vi "Host 9159 cRIO Interface.vi"(10 "Number of Elements":u32=64) -> (2 "AI Data":i32[](array[numeric]))   [LabVIEW 2017]
uses:
  <vilib>/FPGAPlugInAG/NI 9159/niLvFpga_Open_NI 9159.vi
  <vilib>/rvi/interface/common/dynamic/niFpgaDynamicAddResources.vi
  <vilib>/FPGAPlugInAG/Dynamic/niLvFpga_Run_Dynamic.vi
  <vilib>/rvi/interface/common/niFpgaWaitOnOcc.vi
  <vilib>/Utility/error.llb/Error Cluster From Error Code.vi
  <vilib>/rvi/errors/niLvFpgaAdjustHostInterfaceError.vi
  <vilib>/FPGAPlugInAG/Dynamic/niLvFpga_Close_Dynamic.vi
  <vilib>/rvi/interface/nirviOpenFPGA/nirviOpenFPGA.xnode
  FPGA Bitfiles/RIOExpansionLate_FPGATarget2_9159FPGADMATop_ueHRLpdidM4.lvbitx
  FPGA/MXIe 9159 FPGA VI.vi
  <vilib>/rvi/interface/nirviMethod/nirviMethod.xnode
  <vilib>/rvi/interface/nirviReadWriteControl/nirviReadWriteControl.xnode
  <vilib>/rvi/interface/nirviCloseFPGA/nirviCloseFPGA.xnode
  <vilib>/FPGAPlugInAG/Dynamic/niLvFpga_ReadFifo_Dynamic.vi
  <vilib>/rvi/errors/niLvFpgaMergeErrorWithErrorCode.vi
  NiFpgaLv.dll
  <vilib>/rvi/interface/Simulation/niFpgaSimulationCallBeginRW.vi
  <vilib>/FPGAPlugInAG/Dynamic/niLvFpga_ConfigureFifo_Dynamic.vi
panel:
  out "Host Loop Duration (ms)":u32
  out "TargetToHostLoopIterCount":i32
  out "TargetToHostLoopTimedOut":bool
  out "SlowDOLoop_Duration_ticks":u32
  out "FastAILoop_Duration_ticks":u32
  out "Mod3_AI3_I32":i32
  out "Mod3_AI2_I32":i32
  out "Mod3_AI1_I32":i32
  out "Mod3_AI0_I32":i32
  out "SlowScanLoopTimedOut":bool
  out "SlowScanLoop_Duration_ticks":u32
  out "FastDI_U8":u8
  in  "Mod11_U32":u32
  in  "Mod10_U32":u32
  in  "Mod9_U32":u32
  in  "Mod7_U32":u32
  in  "SlowDOLoop_Rate_us":u32=10000
  in  "FastAILoop_Rate_us":u32=1000
  in  "SlowScanLoop_Rate_us":u32=10000
  in  "FastDO_U8":u8
  out "error out":errorcluster={"status"=TRUE, "code"=-50400, "source"="Invoke Method: FIFO.Read in Host 9159 cRIO Interface.vi"}
  in  "stop":bool
  out "Elements Remaining":u32=63
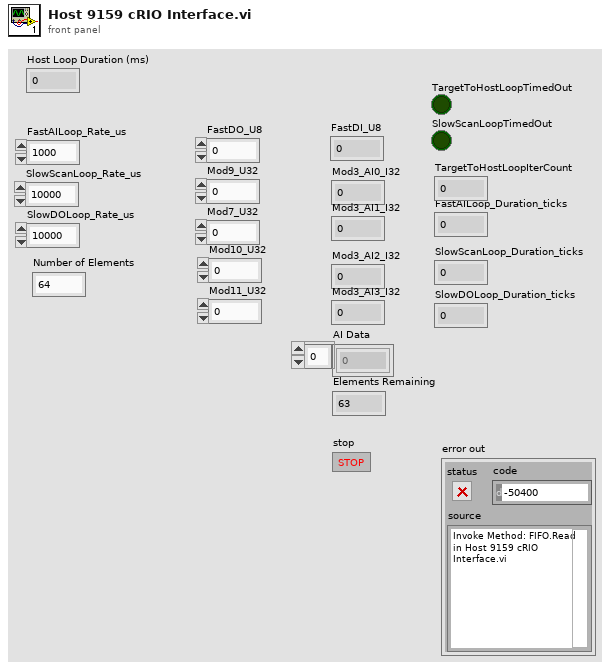
[diagram p1: front panel]
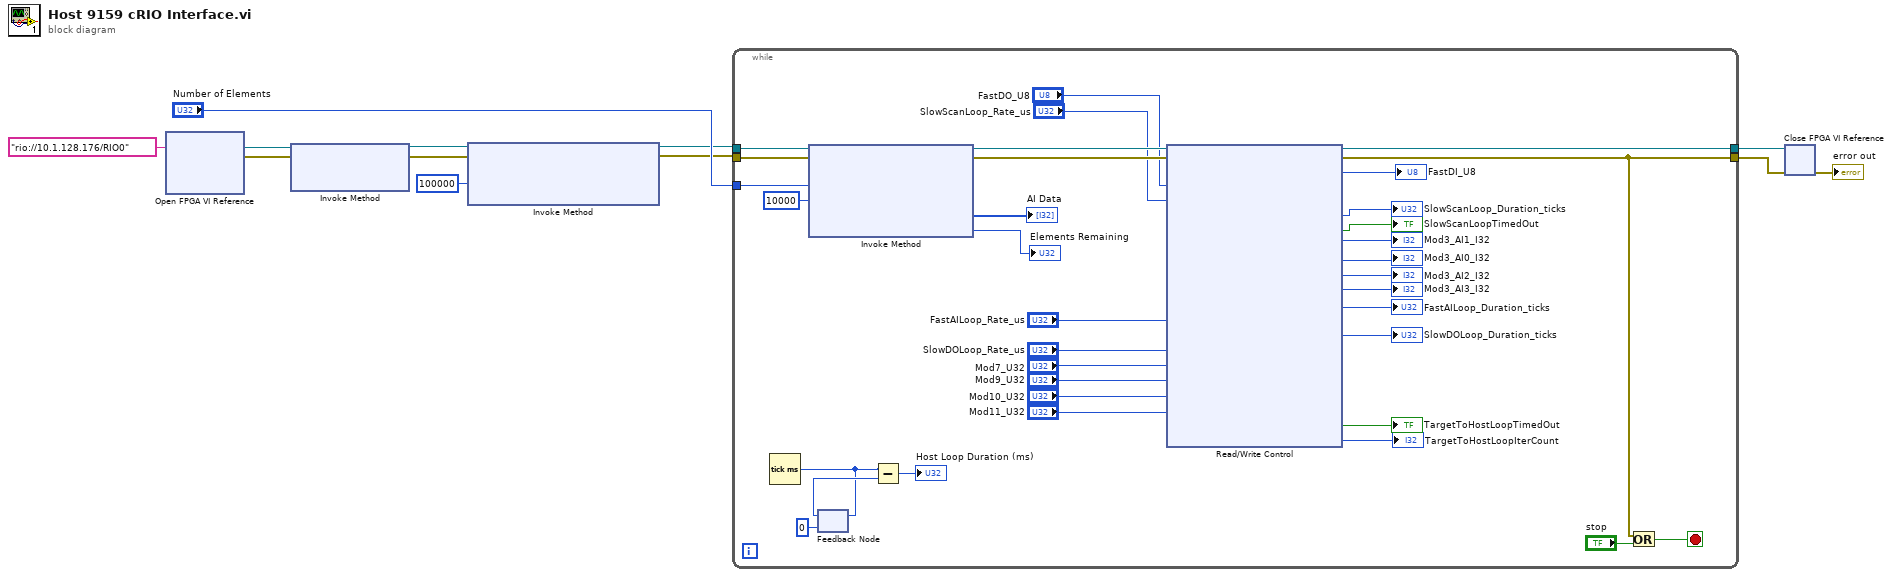
[diagram p0: block diagram]
diagram:
  n1 = xnode "Open FPGA VI Reference"("resource name"=tag "rio://10.1.128.176/RIO0") -> ("FPGA VI Reference Out"=w9:refnum<k20>, "error out"=w8:errorcluster)  [unwired: 1 in]
  n2 = xnode "Invoke Method"("FPGA VI Reference In"=w9, "error in"=w8) -> ("FPGA VI Reference Out"=w5:refnum<k20>, "error out"=w4:errorcluster)  [unwired: 1 in]
  n3 = xnode "Invoke Method"("FPGA VI Reference In"=w5, "error in"=w4, "Requested Depth"=u32 100000) -> ("FPGA VI Reference Out"=w1:refnum<k20>, "error out"=w2:errorcluster)  [unwired: 1 out]
  n4 = while {
    tunnel: w1 -> [w46]
    tunnel: w2 -> [w45]
    tunnel: "Number of Elements" -> [w44]
    tunnel: [w20] -> w7
    tunnel: [w19] -> w6
    stop <- w40 stop-if-true
    n5 = Tick Count (ms)() -> (millisecond timer value=w15:u32)
    n6 = xnode "Invoke Method"("FPGA VI Reference In"=w46, "error in"=w45, "Number of Elements"=w44, "Timeout (ms)"=10000) -> ("FPGA VI Reference Out"=w38:refnum<k20>, "error out"=w37:errorcluster, "Data"=→"AI Data":i32[], "Elements Remaining"=→"Elements Remaining":u32)
    n7 = feedback-in #1(w15) -> ()
    n8 = feedback #1(u32 0 ("millisecond timer value")) -> (w16:u32)
    n9 = Subtract(x=w15, y=w16) -> (x-y=→"Host Loop Duration (ms)":u32)
    n10 = xnode "Read/Write Control"("FPGA VI Reference In"=w38, "error in"=w37, "FastDO_U8"="FastDO_U8", "SlowScanLoop_Rate_us"="SlowScanLoop_Rate_us", "FastAILoop_Rate_us"="FastAILoop_Rate_us", "SlowDOLoop_Rate_us"="SlowDOLoop_Rate_us", "Mod7_U32"="Mod7_U32", "Mod9_U32"="Mod9_U32", "Mod10_U32"="Mod10_U32", "Mod11_U32"="Mod11_U32") -> ("FPGA VI Reference Out"=w20:refnum<k20>, "error out"=w19:errorcluster, "FastDI_U8"=→"FastDI_U8":u8, "SlowScanLoop_Duration_ticks"=→"SlowScanLoop_Duration_ticks":u32, "SlowScanLoopTimedOut"=→"SlowScanLoopTimedOut":bool, "Mod3_AI1_I32"=→"Mod3_AI0_I32" →"Mod3_AI1_I32":i32, "Mod3_AI2_I32"=→"Mod3_AI2_I32":i32, "Mod3_AI3_I32"=→"Mod3_AI3_I32":i32, "FastAILoop_Duration_ticks"=→"FastAILoop_Duration_ticks":u32, "SlowDOLoop_Duration_ticks"=→"SlowDOLoop_Duration_ticks":u32, "TargetToHostLoopTimedOut"=→"TargetToHostLoopTimedOut":bool, "TargetToHostLoopIterCount"=→"TargetToHostLoopIterCount":i32)  [unwired: 1 out]
    n11 = Or(x=w19, y="stop") -> (x .or. y?=w40:bool)
  }
  n12 = xnode "Close FPGA VI Reference"("FPGA VI Reference In"=w7, "error in"=w6) -> ("error out"=→"error out":errorcluster)
